vi "FileIO-Create Folder.vi"(0 "folder":path, 11 "error in (no error)":errorcluster) -> (4 "dup path":path)   [LabVIEW 2020]
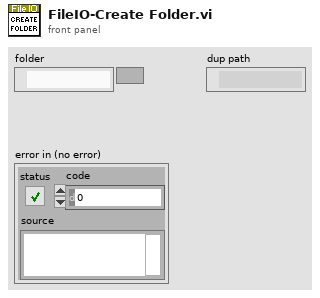
[diagram p1: front panel]
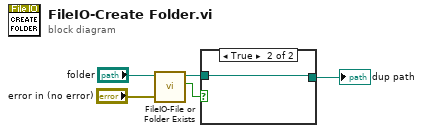
[diagram p0: block diagram]
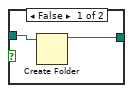
[diagram p2: hidden frame]
diagram:
  n1 = call "FileIO-File or Folder Exists.vi"("error in (no error)"="error in (no error)", "path"="folder") -> ("Directory?"=w3:bool, "dup path"=w4:path)  [unwired: 6 in, 2 out]
  n2 = case shown="True" w3 {
    tunnel: w4 -> [w7 w8]
    tunnel: [w6 w8] -> w5
    frame False {
      n3 = Create Folder(path (use dialog)=w7) -> (created path=w6:path)  [unwired: 2 in, 2 out]
    }
    frame True {
    }
  }
  "dup path" <- w5
